vi "Right Menu Refs.vi"() -> ()   [LabVIEW 2020]
uses:
  Cluster - ATM Machine Data.ctl
  ATM Machine.lvlib
panel:
  out "error out":errorcluster
  in  "error in":errorcluster
  out "ATM Data Out":T1
  in  "ATM Data":T1
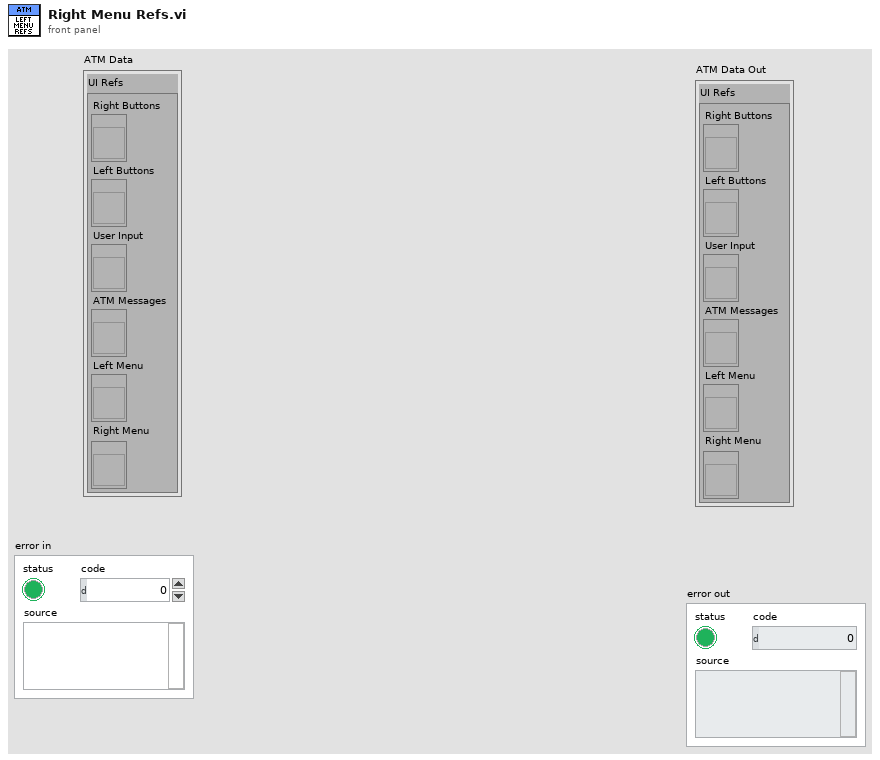
[diagram p1: front panel]
types:
  T1 = typedef "ATM Machine.lvlib/Cluster - ATM Machine Data.ctl" = cluster{"UI Refs":cluster{"Right Buttons":refnum<vi>, "Left Buttons":refnum<vi>, "User Input":refnum<vi>, "ATM Messages":refnum<vi>, "Left Menu":refnum<vi>, "Right Menu":refnum<vi>}}
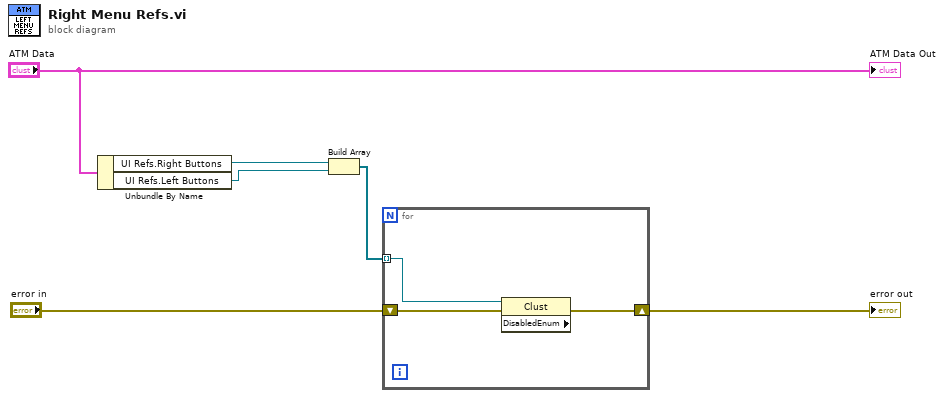
[diagram p0: block diagram]
diagram:
  n1 = Unbundle By Name("ATM Data") -> ("UI Refs.Right Buttons"=w1:refnum<vi>, "UI Refs.Left Buttons"=w5:refnum<vi>)
  n2 = Build Array(w1, w5) -> (w2:refnum<vi>[])
  n3 = for {
    shift-right: [w8] -> w4
    shift-left: "error in" -> [w9]
    tunnel: w2 -> [w7] mode=indexing
    n4 = property class="Clust" props=["DisabledEnum"](reference=w7, error in=w9) -> (error out=w8:errorcluster)  [unwired: 2 out]
  }
  "error out" <- w4
  "ATM Data Out" <- "ATM Data"
